vi "Calculate Robot Heading.vi"(4 "Magnetometer or Gyro used as Robot Angle? (Mag = T, Gyr = F)":bool) -> (0 "Robot Heading":dbl, 1 "Robot Angle":dbl)   [LabVIEW 2014]
uses:
  <vilib>/Rock Robotics/WPI/DriverStation/WPI_DriverStationRobotMode2.ctl
  Global Variables/Sensor Data (Edited).vi
  Global Variables/Miscalleneous.vi
  Robot Global Data.vi
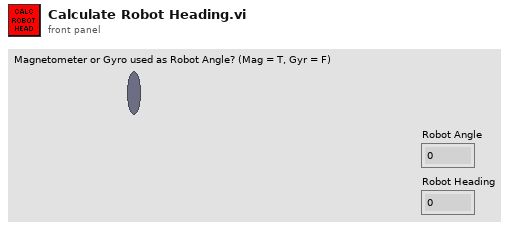
[diagram p1: front panel]
types:
  T1 = typedef "WPI_DriverStationRobotMode2.ctl" = enum16{"Autonomous Disabled", "Autonomous Enabled", "Teleop Disabled", "Teleop Enabled", "Disconnected", "Finish", "Test Disabled", "Test Enabled", "Emergency Stopped"}
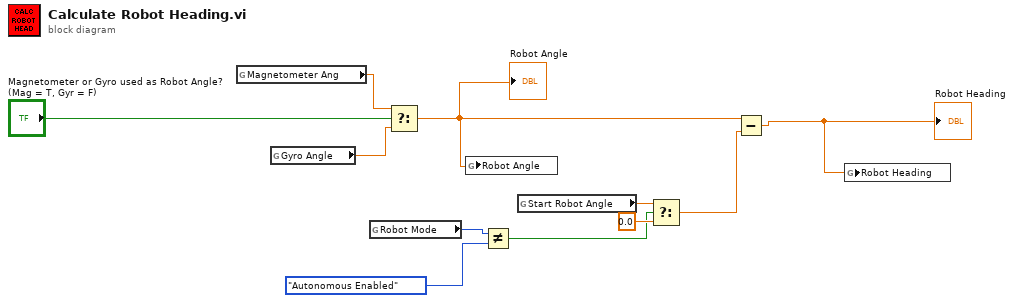
[diagram p0: block diagram]
diagram:
  n1 = global read "Sensor Data (Edited).vi" "Magnetometer Ang"() -> (w9:dbl)
  n2 = global read "Sensor Data (Edited).vi" "Gyro Angle"() -> (w10:dbl)
  n3 = global read "Robot Global Data.vi" "Robot Mode"() -> (w4:T1)
  n4 = Select(t=w9, s="Magnetometer or Gyro used as Robot Angle? (Mag = T, Gyr = F)", f=w10) -> (s? t:f=w7:dbl)
  "Robot Angle" <- w7
  n5 = global write "Sensor Data (Edited).vi" "Robot Angle"(w7) -> ()
  n6 = Not Equal?(x=w4, y=WPI_DriverStationRobotMode2."Autonomous Enabled") -> (x != y?=w2:bool)
  n7 = global read "Miscalleneous.vi" "Start Robot Angle"() -> (w6:dbl)
  n8 = Select(t=w6, s=w2, f=0.0) -> (s? t:f=w1:dbl)
  n9 = Subtract(x=w7, y=w1) -> (x-y=w8:dbl)
  "Robot Heading" <- w8
  n10 = global write "Sensor Data (Edited).vi" "Robot Heading"(w8) -> ()
